vi "BuildInterface.vi"(8 "error in (no error)":errorcluster, 11 "CreateInterface in":refnum<class "CreateInterface.lvclass">) -> (0 "error out":errorcluster, 3 "CreateInterface out":refnum<class "CreateInterface.lvclass">)   [LabVIEW 2020, in "Mermaid.lvlib" / "CreateInterface.lvclass"]
uses:
  CreateInterface.lvclass
  CreateInterface.lvclass/CreateInterface.ctl
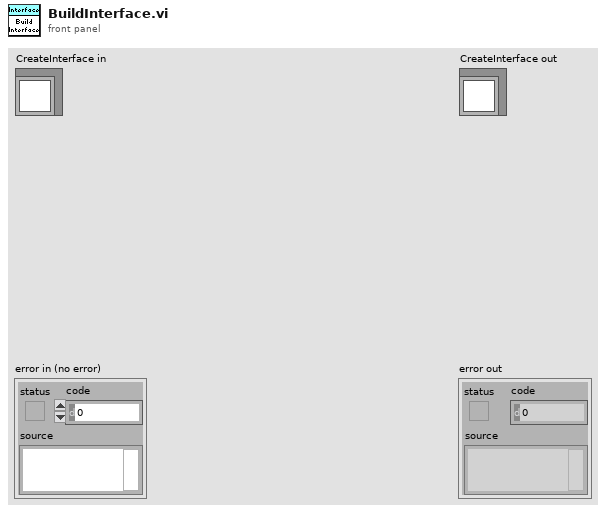
[diagram p1: front panel]
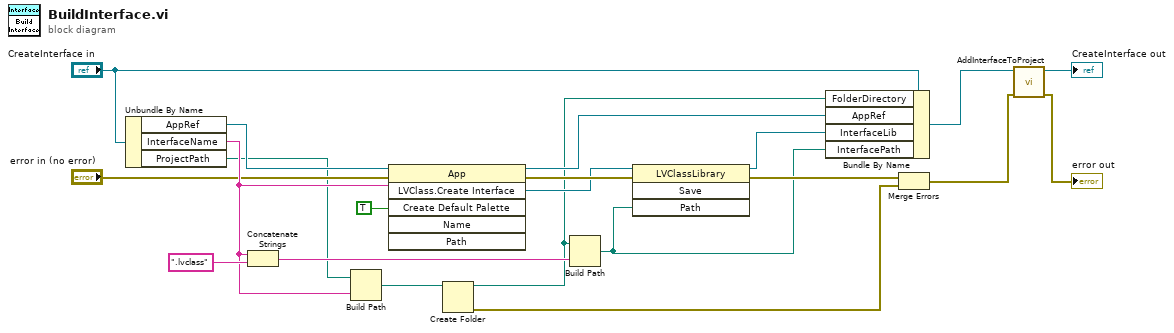
[diagram p0: block diagram]
diagram:
  n1 = Unbundle By Name("CreateInterface in") -> ("AppRef"=w15:refnum<vi>, "InterfaceName"=w14:string, "ProjectPath"=w1:path)
  n2 = Concatenate Strings(w14, ".lvclass" ("string")) -> (w19:string)
  n3 = Build Path(base path=w1, name or relative path=w14) -> (appended path=w17:path)
  n4 = invoke class="App" method="LVClass.Create Interface"(reference=w15, error in="error in (no error)", "Create Default Palette"=TRUE ("Create:Default Palette"), "Name"=w14) -> (reference out=w12:refnum<vi>, error out=w18:errorcluster, "LVClass.Create Interface"=w16:refnum<vi>)  [unwired: 2 in, 3 out]
  n5 = Create Folder(path (use dialog)=w17) -> (created path=w7:path, error out=w8:errorcluster)  [unwired: 2 in, 1 out]
  n6 = Build Path(base path=w7, name or relative path=w19) -> (appended path=w6:path)
  n7 = invoke class="LVClassLibrary" method="Save"(reference=w16, error in=w18, "Path"=w6) -> (reference out=w13:refnum<vi>, error out=w9:errorcluster)  [unwired: 1 in, 2 out]
  n8 = Bundle By Name(cluster="CreateInterface in", "FolderDirectory"=w7, "AppRef"=w12, "InterfaceLib"=w13, "InterfacePath"=w6) -> (w5:refnum<class "CreateInterface.lvclass">)
  n9 = Merge Errors(w9, w8) -> (w3:errorcluster)
  n10 = call "AddInterfaceToProject.vi"("error in (no error)"=w3, "CreateInterface in"=w5) -> ("error out"=→"error out":errorcluster, "CreateInterface out"=→"CreateInterface out":refnum<class "CreateInterface.lvclass">)  [unwired: 8 in]
